vi "test Get Transfer Identifier.vi"(8 "error in":errorcluster, 11 "TestCase in":refnum<class "Engine.lvclass">) -> (0 "error out":errorcluster, 3 "TestCase out":refnum<class "Engine.lvclass">)   [LabVIEW 2024, in "Engine.lvclass"]
uses:
  Engine.lvclass
  Shared/Label.ctl
  <vilib>/addons/_JKI Toolkits/VI Tester/TestCase.llb/TestCase.lvclass
  Hardware API/AIM ARINC 429 Hardware API.lvlib
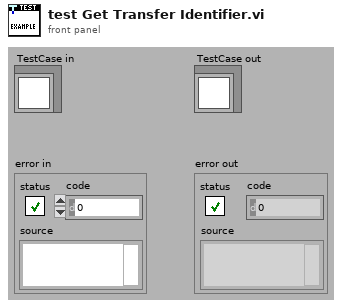
[diagram p1: front panel]
types:
  T1 = typedef "Label.ctl" = u8
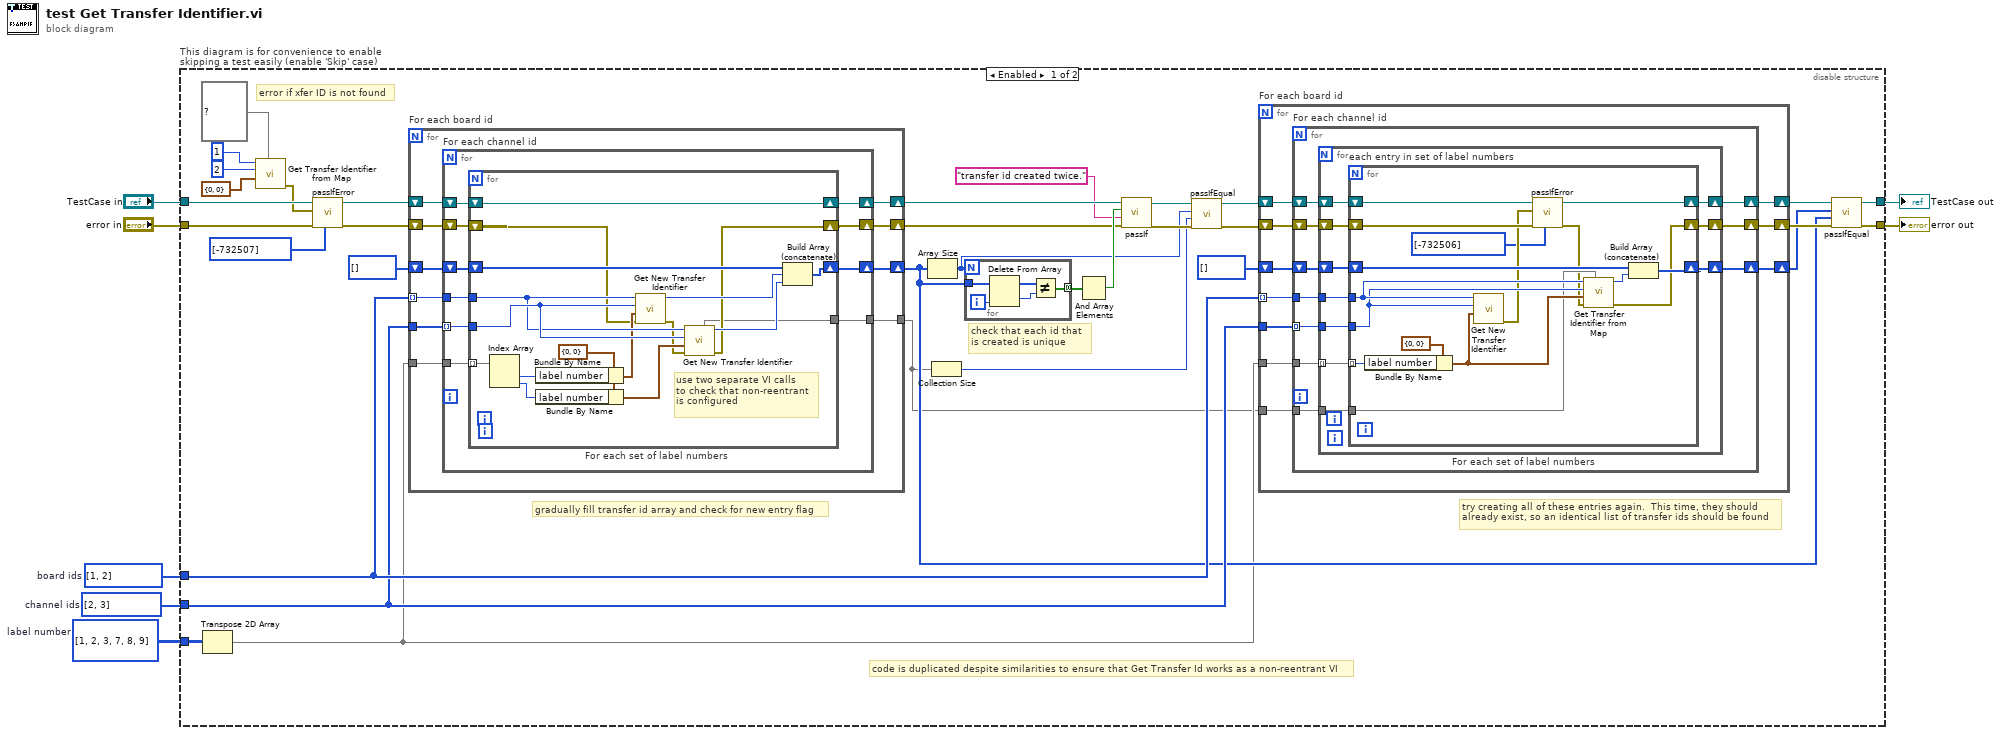
[diagram p0: block diagram]
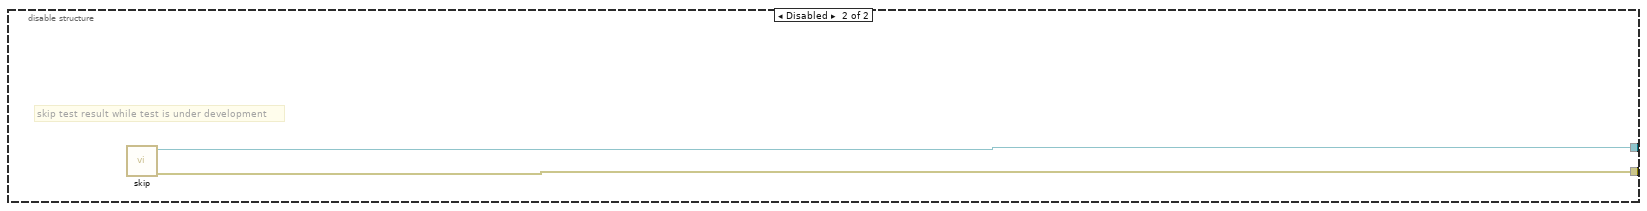
[diagram p2: hidden frame]
diagram:
  w2 = T1[][] [[1, 2, 3], [7, 8, 9]]  # label number
  w1 = u8[] [2, 3]  # channel ids
  w5 = u8[] [1, 2]  # board ids
  n1 = disable-structure "This diagram is for convenience to enable skipping a test easily (enable 'Skip' case)" shown="Enabled" {
    disable-tunnel: [w32 w131] -> w6
    disable-tunnel: [w34 w132] -> w7
    disable-tunnel: w5 -> [w37 _]
    disable-tunnel: "error in" -> [w23 _]
    disable-tunnel: "TestCase in" -> [w22 _]
    disable-tunnel: w2 -> [w16 _]
    disable-tunnel: w1 -> [w36 _]
    frame Enabled {
      # "error if xfer ID is not found"
      # "code is duplicated despite similarities to ensure that Get Transfer Id works as a non-reentrant VI"
      # "try creating all of these entries again.  This time, they should\nalready exist, so an identical list of transfer ids should be found"
      # "check that each id that \nis created is unique"
      # "gradually fill transfer id array and check for new entry flag"
      n2 = Transpose 2D Array(2D array=w16) -> (transposed array=w15:T1[][])
      n3 = call "Get Transfer Identifier from Map.vi"("Transfer ID map"=map{u32, u32} {}, "label information"=cluster{"label number":T1, "sdi":u8} {"label number"=0, "sdi"=0}, "channel number in"=u8 2, "board number in"=u8 1) -> ("error out"=w18:errorcluster)  [unwired: 6 in, 1 out]
      n4 = call-dynamic "passIfError.vi"("passing error codes (default = any error code)"=i32[] [-732507], "error in (no error)"=w23, "error"=w18, "TestCase in"=w22) -> ("error out"=w20:errorcluster, "TestCase out"=w21:refnum<class "Engine.lvclass">)  [unwired: 6 in]
      n5 = for "For each board id" {
        tunnel: w37 -> [w51] mode=indexing
        shift-right: [w47] -> w39
        shift-left: w20 -> [w48]
        shift-right: [w49] -> w38
        shift-left: w21 -> [w50]
        shift-right: [w43] -> w27
        shift-left: u32[] [] ("created xfer ids \npart 1") -> [w46]
        tunnel: w15 -> [w45]
        tunnel: w36 -> [w44]
        tunnel: [w42] -> w14
        n6 = for "For each channel id" {
          tunnel: w51 -> [w54]
          shift-right: [w58] -> w47
          shift-left: w48 -> [w60]
          shift-right: [w59] -> w49
          shift-left: w50 -> [w61]
          shift-right: [w53] -> w43
          shift-left: w46 -> [w57]
          tunnel: w45 -> [w56]
          tunnel: w44 -> [w55] mode=indexing
          tunnel: [w52] -> w42
          n7 = for "For each set of label numbers" {
            shift-right: [w64] -> w58
            shift-left: w60 -> [w65]
            shift-right: [w78] -> w59
            shift-left: w61 -> [w78]
            shift-right: [w73] -> w53
            shift-left: w57 -> [w74]
            tunnel: w56 -> [w77] mode=indexing
            tunnel: w55 -> [w76]
            tunnel: w54 -> [w75]
            tunnel: [w62] -> w52
            w68 = cluster{"label number":T1, "sdi":u8} {"label number"=0, "sdi"=0} ("label information")
            # "use two separate VI calls \nto check that non-reentrant\nis configured"
            n8 = Index Array(array=w77) -> (element #1=w70:T1, element #2=w69:T1)  [unwired: 2 in]
            n9 = Bundle By Name(cluster=w68, "label number"=w70) -> (w67:cluster{"label number":T1, "sdi":u8})
            n10 = Bundle By Name(cluster=w68, "label number"=w69) -> (w66:cluster{"label number":T1, "sdi":u8})
            n11 = call "Get New Transfer Identifier.vi"("error in"=w65, "label information"=w67, "channel number in"=w76, "board number in"=w75) -> ("error out"=w63:errorcluster, "Transfer ID out"=w72:u32)  [unwired: 5 in, 1 out]
            n12 = call "Get New Transfer Identifier.vi"("error in"=w63, "label information"=w66, "channel number in"=w76, "board number in"=w75) -> ("error out"=w64:errorcluster, "Transfer ID out"=w71:u32, "Transfer ID map"=w62:map{u32, u32})  [unwired: 5 in]
            n13 = Build Array (concatenate)(w74, w72, w71) -> (w73:u32[])
          }
        }
      }
      n14 = Array Size(array=w27) -> (size(s)=w8:i32)
      n15 = Collection Size(1:w14) -> (0:w9:i32)
      n16 = for {
        N: w8 -> [_]
        tunnel: [w83] -> w40 mode=concatenating
        tunnel: w27 -> [w81]
        i -> [w82]
        n17 = Delete From Array(array=w81, index=w82) -> (deleted portion=w79:u32, array with subset deleted=w80:u32[])  [unwired: 1 in]
        n18 = Not Equal?(x=w80, y=w79) -> (x != y?=w83:bool[])
      }
      n19 = And Array Elements(Boolean array=w40) -> (logical AND=w41:bool)
      n20 = call-dynamic "passIf.vi"("error in (no error)"=w39, "message (\"\")"="transfer id created twice." ("message (\"\")"), "pass"=w41, "TestCase in"=w38) -> ("error out"=w10:errorcluster, "TestCase out"=w13:refnum<class "Engine.lvclass">)  [unwired: 6 in]
      n21 = call-dynamic "passIfEqual.vi"("error in (no error)"=w10, "y"=w9, "x"=w8, "TestCase in"=w13) -> ("error out"=w11:errorcluster, "TestCase out"=w12:refnum<class "Engine.lvclass">)  [unwired: 6 in]
      n22 = for "For each board id" {
        tunnel: w37 -> [w93] mode=indexing
        shift-right: [w89] -> w35
        shift-left: w11 -> [w90]
        shift-right: [w91] -> w33
        shift-left: w12 -> [w92]
        shift-right: [w85] -> w29
        shift-left: u32[] [] ("created xfer ids \npart 2") -> [w88]
        tunnel: w15 -> [w87]
        tunnel: w36 -> [w86]
        tunnel: w14 -> [w84]
        n23 = for "For each channel id" {
          tunnel: w93 -> [w96]
          shift-right: [w100] -> w89
          shift-left: w90 -> [w102]
          shift-right: [w101] -> w91
          shift-left: w92 -> [w103]
          shift-right: [w95] -> w85
          shift-left: w88 -> [w99]
          tunnel: w87 -> [w98]
          tunnel: w86 -> [w97] mode=indexing
          tunnel: w84 -> [w94]
          n24 = for "For each set of label numbers" {
            shift-right: [w108] -> w100
            shift-left: w102 -> [w105]
            shift-right: [w109] -> w101
            shift-left: w103 -> [w113]
            shift-right: [w106] -> w95
            shift-left: w99 -> [w107]
            tunnel: w98 -> [w112] mode=indexing
            tunnel: w97 -> [w111]
            tunnel: w96 -> [w110]
            tunnel: w94 -> [w104]
            n25 = for "each entry in set of label numbers" {
              tunnel: w112 -> [w126] mode=indexing
              tunnel: w111 -> [w124]
              tunnel: w110 -> [w125]
              shift-right: [w117] -> w109
              shift-left: w113 -> [w118]
              shift-right: [w115] -> w108
              shift-left: w105 -> [w120]
              shift-right: [w128] -> w106
              shift-left: w107 -> [w129]
              tunnel: w104 -> [w121]
              n26 = Bundle By Name(cluster=cluster{"label number":T1, "sdi":u8} {"label number"=0, "sdi"=0} ("label information"), "label number"=w126) -> (w123:cluster{"label number":T1, "sdi":u8})
              n27 = call "Get New Transfer Identifier.vi"("label information"=w123, "channel number in"=w124, "board number in"=w125) -> ("error out"=w119:errorcluster)  [unwired: 6 in, 2 out]
              n28 = call-dynamic "passIfError.vi"("passing error codes (default = any error code)"=i32[] [-732506], "error in (no error)"=w120, "error"=w119, "TestCase in"=w118) -> ("error out"=w116:errorcluster, "TestCase out"=w117:refnum<class "Engine.lvclass">)  [unwired: 6 in]
              n29 = call "Get Transfer Identifier from Map.vi"("Transfer ID map"=w121, "error in"=w116, "label information"=w123, "channel number in"=w124, "board number in"=w125) -> ("error out"=w115:errorcluster, "Transfer ID out"=w122:u32)  [unwired: 5 in]
              n30 = Build Array (concatenate)(w129, w122) -> (w128:u32[])
            }
          }
        }
      }
      n31 = call-dynamic "passIfEqual.vi"("error in (no error)"=w35, "y"=w27, "x"=w29, "TestCase in"=w33) -> ("error out"=w34:errorcluster, "TestCase out"=w32:refnum<class "Engine.lvclass">)  [unwired: 6 in]
    }
    frame Disabled {
      # "skip test result while test is under development"
      n32 = call <vilib>:"skip.vi"() -> ("error out"=w132:errorcluster, "TestCase out"=w131:refnum<class "Engine.lvclass">, "error in (no error)"=w130:errorcluster, "TestCase in"=w133:refnum<class "Engine.lvclass">)  [unwired: 8 in]
    }
  }
  "error out" <- w7
  "TestCase out" <- w6
